vi "Source_Q_wrong.vi"(2 "Ch Names":string[](array[string]), 3 "Values":dbl[](array[numeric]) format="%.2f") -> (0 "Gas Error?":bool)   [LabVIEW 2013]
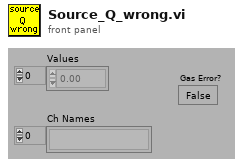
[diagram p1: front panel]
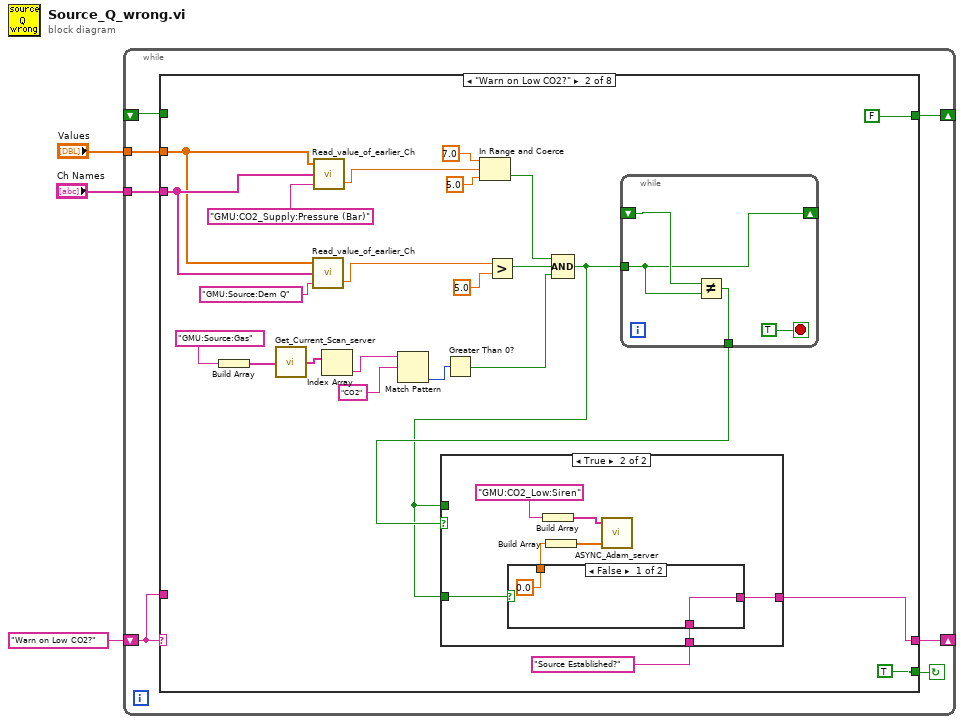
[diagram p0: block diagram]
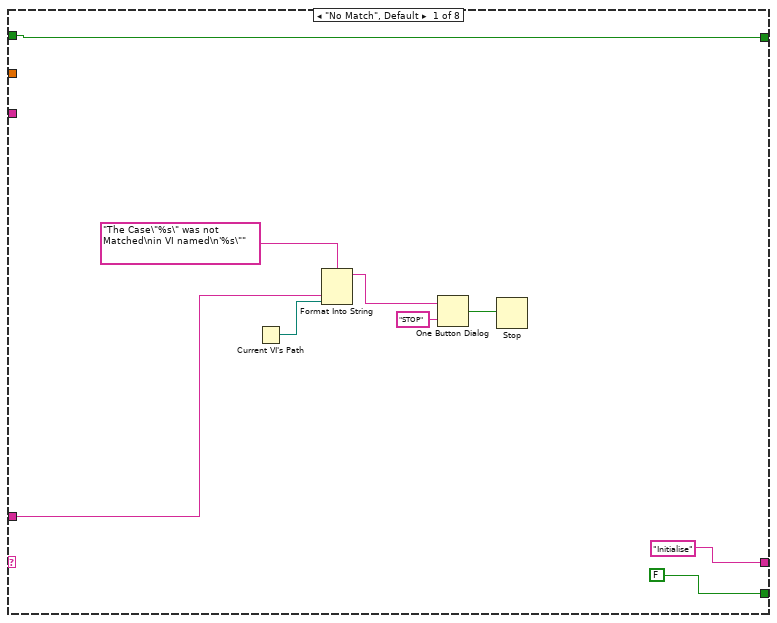
[diagram p2: hidden frame]
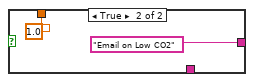
[diagram p4: hidden frame]
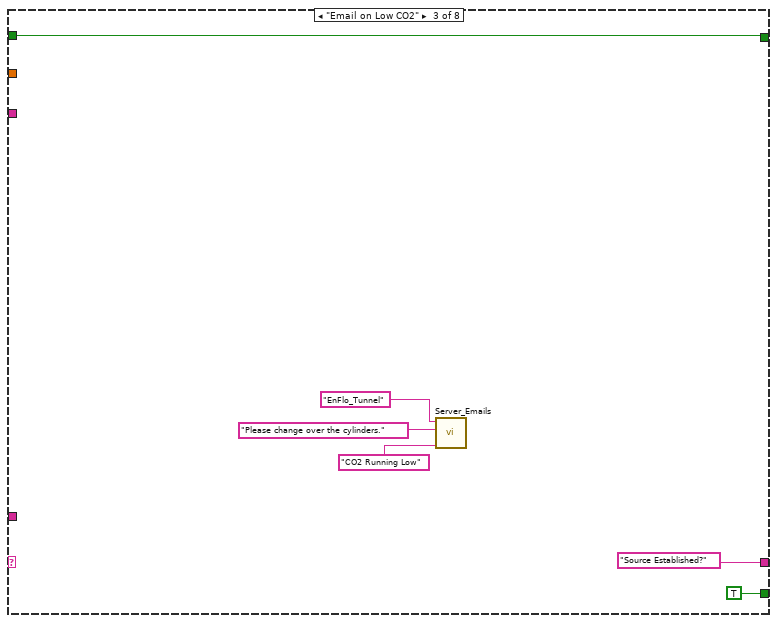
[diagram p5: hidden frame]
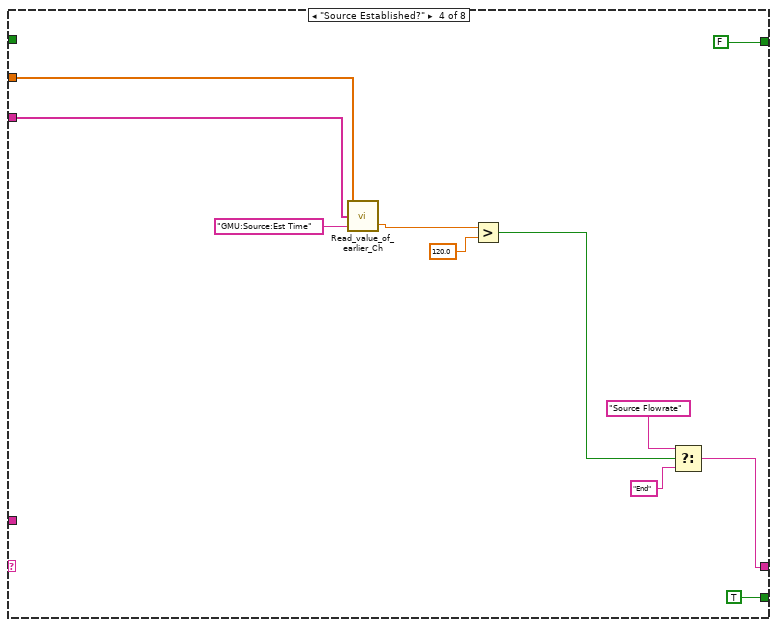
[diagram p6: hidden frame]
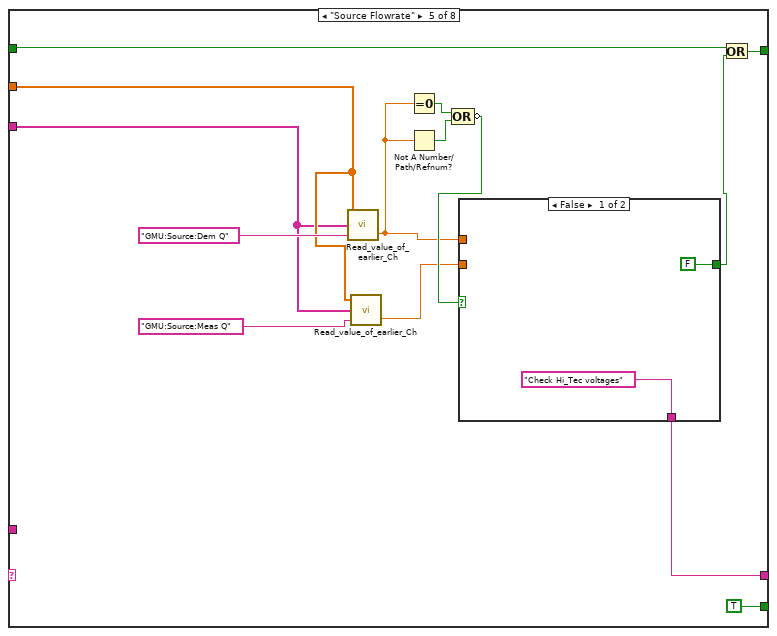
[diagram p7: hidden frame]
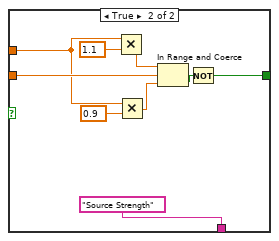
[diagram p8: hidden frame]
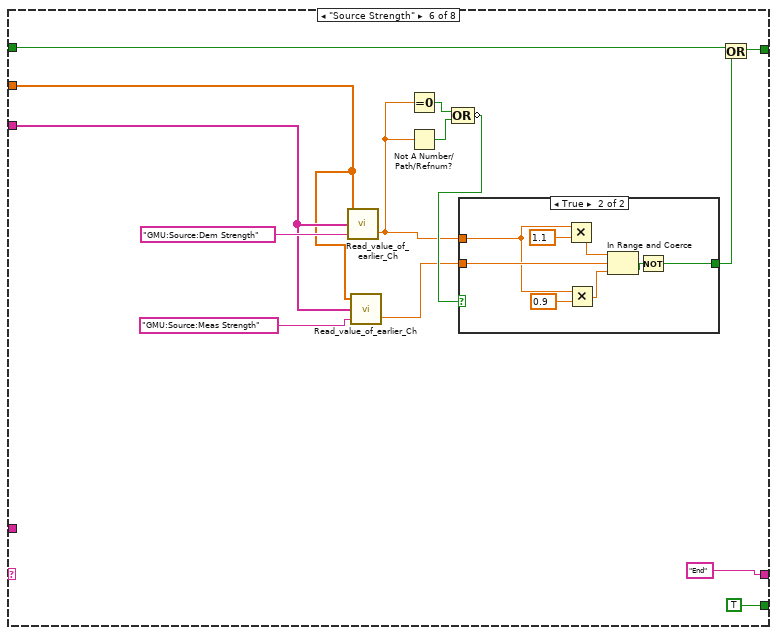
[diagram p9: hidden frame]
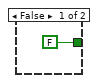
[diagram p10: hidden frame]
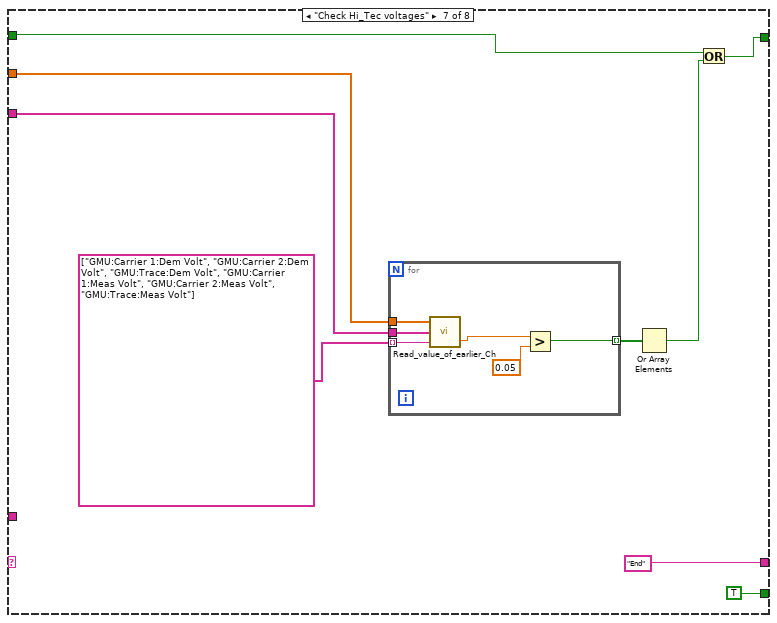
[diagram p11: hidden frame]
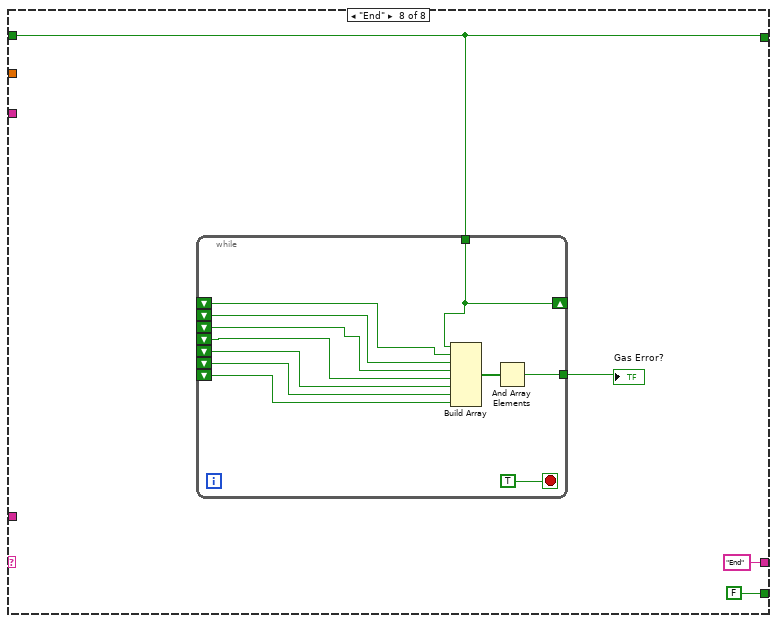
[diagram p12: hidden frame]
diagram:
  n1 = while {
    shift-left: "Warn on Low CO2?" -> [w8]
    shift-right: [w9] -> _
    tunnel: "Ch Names" -> [w7]
    tunnel: "Values" -> [w6]
    shift-right: [w5] -> _
    shift-left: _ -> [w4]
    stop <- w10 continue-if-true
    n2 = case shown="\"Warn on Low CO2?\"" w8 {
      tunnel: [FALSE TRUE TRUE TRUE TRUE TRUE TRUE FALSE] -> w10
      tunnel: ["Initialise" w28 "Source Established?" w67 w77 "End" ("f") "End" "End" ("f")] -> w9
      tunnel: w8 -> [w14 _ _ _ _ _ _ _]
      tunnel: w7 -> [_ w37 _ w75 w88 w104 w131 _]
      tunnel: w6 -> [_ w36 _ w74 w89 w103 w129 _]
      tunnel: [w11 FALSE w64 FALSE w80 w105 w125 w141] -> w5
      tunnel: w4 -> [w11 _ w64 _ w78 w106 w126 w141]
      frame "No Match", Default {
        n3 = Current VI's Path() -> (path=w13:path)
        n4 = Format Into String(format string="The Case\"%s\" was not Matched\nin VI named\n'%s\"" ("Format String"), w14, w13) -> (resulting string=w17:string)  [unwired: 2 in, 1 out]
        n5 = One Button Dialog(message=w17, button name ("OK")="STOP") -> (true=w15:bool)
        n6 = Stop(stop? (T)=w15) -> ()
      }
      frame "Warn on Low CO2?" {
        n7 = Build Array("GMU:Source:Gas") -> (w25:string[])
        n8 = call "Get_Current_Scan_server.vi"("Desired Channels"=w25) -> ("String values"=w24:string[])  [unwired: 2 out]
        n9 = call "Read_value_of_earlier_Ch.vi"("Desired Ch to Read"="GMU:Source:Dem Q", "Ch names"=w37, "Present scan array"=w36) -> ("Value"=w34:dbl)  [unwired: 1 in, 1 out]
        n10 = call "Read_value_of_earlier_Ch.vi"("Desired Ch to Read"="GMU:CO2_Supply:Pressure (Bar)", "Ch names"=w37, "Present scan array"=w36) -> ("Value"=w35:dbl)  [unwired: 1 in, 1 out]
        n11 = Index Array(array=w24) -> (element=w23:string)  [unwired: 1 in]
        n12 = Match Pattern(string=w23, regular expression="CO2") -> (offset past match=w21:i32)  [unwired: 1 in, 3 out]
        n13 = Greater Than 0?(x=w21) -> (x > 0?=w20:bool)
        n14 = In Range and Coerce(upper limit=7.0, x=w35, lower limit=5.0) -> (In Range?=w32:bool)  [unwired: 1 out]
        n15 = Greater?(x=w34, y=5.0) -> (0:w31:bool)
        n16 = Compound Arithmetic op=AND(w32, w31, w20) -> (w29:bool)
        n17 = while {
          shift-right: [w57] -> _
          shift-left: _ -> [w58]
          tunnel: w29 -> [w57]
          tunnel: [w56] -> w30
          stop <- TRUE stop-if-true
          n18 = Not Equal?(x=w58, y=w57) -> (x != y?=w56:bool)
        }
        n19 = case shown="True" w30 {
          tunnel: w29 -> [_ _]
          tunnel: w29 -> [_ w48]
          tunnel: [w44 w46] -> w28
          tunnel: "Source Established?" -> [w44 w45]
          frame False {
          }
          frame True {
            n20 = case shown="False" w48 {
              tunnel: [0.0 ("element") 1.0 ("t")] -> w47
              tunnel: [w52 "Email on Low CO2"] -> w46
              tunnel: w45 -> [w52 _]
              frame False {
              }
              frame True {
              }
            }
            n21 = Build Array("GMU:CO2_Low:Siren") -> (w51:string[])
            n22 = Build Array(w47) -> (w50:dbl[])
            n23 = call "ASYNC_Adam_server.vi"("Values"=w50, "Channel Names"=w51) -> ()  [unwired: 1 in, 3 out]
          }
        }
      }
      frame "Email on Low CO2" {
        n24 = call "Server_Emails.vi"("Client Name Contains"="EnFlo_Tunnel", "Message"="Please change over the cylinders.", "Subject"="CO2 Running Low") -> ()  [unwired: 2 in, 3 out]
      }
      frame "Source Established?" {
        n25 = call "Read_value_of_earlier_Ch.vi"("Desired Ch to Read"="GMU:Source:Est Time", "Ch names"=w75, "Present scan array"=w74) -> ("Value"=w72:dbl)  [unwired: 1 in, 1 out]
        n26 = Greater?(x=w72, y=120.0) -> (0:w69:bool)
        n27 = Select(t="Source Flowrate", s=w69, f="End") -> (s? t:f=w67:string)
      }
      frame "Source Flowrate" {
        n28 = call "Read_value_of_earlier_Ch.vi"("Desired Ch to Read"="GMU:Source:Dem Q", "Ch names"=w88, "Present scan array"=w89) -> ("Value"=w83:dbl)  [unwired: 1 in, 1 out]
        n29 = call "Read_value_of_earlier_Ch.vi"("Desired Ch to Read"="GMU:Source:Meas Q", "Ch names"=w88, "Present scan array"=w89) -> ("Value"=w82:dbl)  [unwired: 1 in, 1 out]
        n30 = Equal To 0?(x=w83) -> (x = 0?=w86:bool)
        n31 = Not A Number/Path/Refnum?(number/path/refnum=w83) -> (NaN/Path/Refnum?=w85:bool)
        n32 = Compound Arithmetic op=OR(w86, w85) -> (invert w84:bool)
        n33 = case shown="False" w84 {
          tunnel: w82 -> [_ w97]
          tunnel: w83 -> [_ w96]
          tunnel: [FALSE w94] -> w79
          tunnel: ["Check Hi_Tec voltages" "Source Strength"] -> w77
          frame False {
          }
          frame True {
            n34 = Multiply(x=w96, y=1.1) -> (x*y=w101:dbl)
            n35 = Multiply(x=w96, y=0.9) -> (x*y=w100:dbl)
            n36 = In Range and Coerce(upper limit=w101, x=w97, lower limit=w100) -> (In Range?=w95:bool)  [unwired: 1 out]
            n37 = Not(x=w95) -> (.not. x?=w94:bool)
          }
        }
        n38 = Or(x=w78, y=w79) -> (x .or. y?=w80:bool)
      }
      frame "Source Strength" {
        n39 = call "Read_value_of_earlier_Ch.vi"("Desired Ch to Read"="GMU:Source:Dem Strength", "Ch names"=w104, "Present scan array"=w103) -> ("Value"=w110:dbl)  [unwired: 1 in, 1 out]
        n40 = call "Read_value_of_earlier_Ch.vi"("Desired Ch to Read"="GMU:Source:Meas Strength", "Ch names"=w104, "Present scan array"=w103) -> ("Value"=w109:dbl)  [unwired: 1 in, 1 out]
        n41 = Equal To 0?(x=w110) -> (x = 0?=w113:bool)
        n42 = Not A Number/Path/Refnum?(number/path/refnum=w110) -> (NaN/Path/Refnum?=w112:bool)
        n43 = Compound Arithmetic op=OR(w113, w112) -> (invert w111:bool)
        n44 = case shown="True" w111 {
          tunnel: w109 -> [_ w120]
          tunnel: w110 -> [_ w119]
          tunnel: [FALSE w117] -> w107
          frame False {
          }
          frame True {
            n45 = Multiply(x=w119, y=1.1) -> (x*y=w124:dbl)
            n46 = Multiply(x=w119, y=0.9) -> (x*y=w123:dbl)
            n47 = In Range and Coerce(upper limit=w124, x=w120, lower limit=w123) -> (In Range?=w118:bool)  [unwired: 1 out]
            n48 = Not(x=w118) -> (.not. x?=w117:bool)
          }
        }
        n49 = Or(x=w106, y=w107) -> (x .or. y?=w105:bool)
      }
      frame "Check Hi_Tec voltages" {
        n50 = for {
          tunnel: w129 -> [w139]
          tunnel: w131 -> [w138]
          tunnel: string[] ["GMU:Carrier 1:Dem Volt", "GMU:Carrier 2:Dem Volt", "GMU:Trace:Dem Volt", "GMU:Carrier 1:Meas Volt", "GMU:Carrier 2:Meas Volt", "GMU:Trace:Meas Volt"] ("appended array") -> [w137] mode=indexing
          tunnel: [w134] -> w128 mode=indexing
          n51 = call "Read_value_of_earlier_Ch.vi"("Desired Ch to Read"=w137, "Ch names"=w138, "Present scan array"=w139) -> ("Value"=w135:dbl)  [unwired: 1 in, 1 out]
          n52 = Greater?(x=w135, y=0.05) -> (0:w134:bool)
        }
        n53 = Or Array Elements(Boolean array=w128) -> (logical OR=w127:bool)
        n54 = Or(x=w126, y=w127) -> (x .or. y?=w125:bool)
      }
      frame "End" {
        n55 = while {
          shift-right: [w153] -> _
          shift-left: _ -> [w152]
          shift-left: _ -> [w151]
          shift-left: _ -> [w150]
          shift-left: _ -> [w149]
          shift-left: _ -> [w148]
          shift-left: _ -> [w147]
          shift-left: _ -> [w146]
          tunnel: w141 -> [w153]
          tunnel: [w144] -> w143
          stop <- TRUE stop-if-true
          n56 = Build Array(w153, w152, w151, w150, w149, w148, w147, w146) -> (w145:bool[])
          n57 = And Array Elements(Boolean array=w145) -> (logical AND=w144:bool)
        }
        "Gas Error?" <- w143
      }
    }
  }
